vi "Read and Write Controls to Automatic Config File.vi"(5 "file name":string, 7 "Action":T1, 8 "error in":errorcluster, 10 "Control References":refnum<vi>[](array[refnum])) -> (0 "error out":errorcluster)   [LabVIEW 2021]
doc: "Writes the values of an array of controls to a configuration file or reads them back.\n<b>Control References</b> is an array of the references of the controls to be saved.\n\nThe configuration file is named after the VI the first control in the array is in and is saved in the LabVIEW Data folder"
uses:
  RWC_Actions.ctl
  <vilib>/Utility/config.llb/NI_LVConfig.lvlib
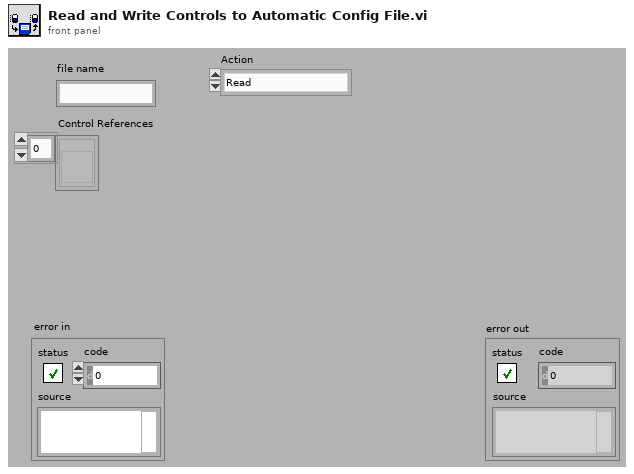
[diagram p1: front panel]
types:
  T1 = typedef "RWC_Actions.ctl" = enum16{"Read", "Write", "Read and Create"}
  T2 = typedef "NI_LVConfig.lvlib/Config Data RefNum.ctl" = refnum<k1>
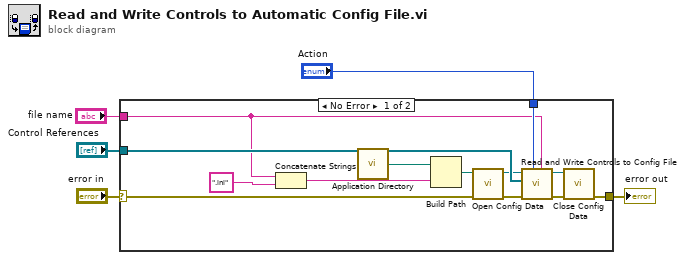
[diagram p0: block diagram]
diagram:
  n1 = case shown="No Error" "error in" {
    selector: "error in" -> [w9 w19]
    tunnel: "Action" -> [w18 _]
    tunnel: "Control References" -> [w17 _]
    tunnel: [w12 w19] -> w2
    tunnel: "file name" -> [w8 _]
    frame No Error {
      n2 = Concatenate Strings(w8, ".ini" ("string")) -> (w6:string)
      n3 = call <vilib>:"Application Directory.vi"() -> ("Application Directory"=w10:path)
      n4 = Build Path(base path=w10, name or relative path=w6) -> (appended path=w11:path)
      n5 = call <vilib>:"Open Config Data.vi"("error in (no error)"=w9, "configuration file path"=w11) -> ("error out"=w16:errorcluster, "refnum"=w14:T2)  [unwired: 7 in, 1 out]
      n6 = call "Read and Write Controls to Config File.vi"("section (optional)"=w8, "Action"=w18, "error in"=w16, "Control References"=w17, "Configuration File Reference In"=w14) -> ("error out"=w13:errorcluster, "Configuration File Reference Out"=w15:T2)  [unwired: 5 in]
      n7 = call <vilib>:"Close Config Data.vi"("error in (no error)"=w13, "refnum"=w15) -> ("error out"=w12:errorcluster)  [unwired: 8 in, 1 out]
    }
    frame Error {
    }
  }
  "error out" <- w2
